vi "Read-Write Config File.vi"(0 "configuration file path":path=path "C:/ProgramData/PVI Systems/Vision Inspection System/Config.ini", 1 "Main Config in":T1 {"OPC Module Configs"."Data"."Variable Array"."status" items=["Good"=0, "Good_SubscriptionTransferred"=2949120, "Good_CompletesAsynchronously"=3014656, "Good_Overload"=3080192, "Good_Clamped"=3145728, "Good_LocalOverride"=9830400, "Good_EntryInserted"=10616832, "Good_EntryReplaced"=10682368, "Good_NoData"=10813440, "Good_MoreData"=10878976, "Good_CommunicationEvent"=10944512, "Good_ShutdownEvent"=11010048, "Good_CallAgain"=11075584, "Good_NonCriticalTimeout"=11141120, "Good_ResultsMayBeIncomplete"=12189696, "Good_DataIgnored"=14221312, "Uncertain"=1073741824, "Uncertain_ReferenceOutOfServer"=1080819712, "Uncertain_NoCommunicationLastUsableValue"=1083113472, "Uncertain_LastUsableValue"=1083179008, "Uncertain_SubstituteValue"=1083244544, "Uncertain_InitialValue"=1083310080, "Uncertain_SensorNotAccurate"=1083375616, "Uncertain_EngineeringUnitsExceeded"=1083441152, "Uncertain_SubNormal"=1083506688, "Uncertain_DataSubNormal"=1084489728, "Uncertain_ReferenceNotDeleted"=1086062592, "Uncertain_NotAllNodesAvailable"=1086324736, "Bad"=2147483648, "Bad_UnexpectedError"=2147549184, "Bad_InternalError"=2147614720, "Bad_OutOfMemory"=2147680256, "Bad_ResourceUnavailable"=2147745792, "Bad_CommunicationError"=2147811328, "Bad_EncodingError"=2147876864, "Bad_DecodingError"=2147942400, "Bad_EncodingLimitsExceeded"=2148007936, "Bad_UnknownResponse"=2148073472, "Bad_Timeout"=2148139008, "Bad_ServiceUnsupported"=2148204544, "Bad_Shutdown"=2148270080, "Bad_ServerNotConnected"=2148335616, "Bad_ServerHalted"=2148401152, "Bad_NothingToDo"=2148466688, "Bad_TooManyOperations"=2148532224, "Bad_DataTypeIdUnknown"=2148597760, "Bad_CertificateInvalid"=2148663296, "Bad_SecurityChecksFailed"=2148728832, "Bad_CertificateTimeInvalid"=2148794368, "Bad_CertificateIssuerTimeInvalid"=2148859904, "Bad_CertificateHostNameInvalid"=2148925440, "Bad_CertificateUriInvalid"=2148990976, "Bad_CertificateUseNotAllowed"=2149056512, "Bad_CertificateIssuerUseNotAllowed"=2149122048, "Bad_CertificateUntrusted"=2149187584, "Bad_CertificateRevocationUnknown"=2149253120, "Bad_CertificateIssuerRevocationUnknown"=2149318656, "Bad_CertificateRevoked"=2149384192, "Bad_CertificateIssuerRevoked"=2149449728, "Bad_UserAccessDenied"=2149515264, "Bad_IdentityTokenInvalid"=2149580800, "Bad_IdentityTokenRejected"=2149646336, "Bad_SecureChannelIdInvalid"=2149711872, "Bad_InvalidTimestamp"=2149777408, "Bad_NonceInvalid"=2149842944, "Bad_SessionIdInvalid"=2149908480, "Bad_SessionClosed"=2149974016, "Bad_SessionNotActivated"=2150039552, "Bad_SubscriptionIdInvalid"=2150105088, "Bad_RequestHeaderInvalid"=2150236160, "Bad_TimestampsToReturnInvalid"=2150301696, "Bad_RequestCancelledByClient"=2150367232, "Bad_NoCommunication"=2150694912, "Bad_WaitingForInitialData"=2150760448, "Bad_NodeIdInvalid"=2150825984, "Bad_NodeIdUnknown"=2150891520, "Bad_AttributeIdInvalid"=2150957056, "Bad_IndexRangeInvalid"=2151022592, "Bad_IndexRangeNoData"=2151088128, "Bad_DataEncodingInvalid"=2151153664, "Bad_DataEncodingUnsupported"=2151219200, "Bad_NotReadable"=2151284736, "Bad_NotWritable"=2151350272, "Bad_OutOfRange"=2151415808, "Bad_NotSupported"=2151481344, "Bad_NotFound"=2151546880, "Bad_ObjectDeleted"=2151612416, "Bad_NotImplemented"=2151677952, "Bad_MonitoringModeInvalid"=2151743488, "Bad_MonitoredItemIdInvalid"=2151809024, "Bad_MonitoredItemFilterInvalid"=2151874560, "Bad_MonitoredItemFilterUnsupported"=2151940096, "Bad_FilterNotAllowed"=2152005632, "Bad_StructureMissing"=2152071168, "Bad_EventFilterInvalid"=2152136704, "Bad_ContentFilterInvalid"=2152202240, "Bad_FilterOperandInvalid"=2152267776, "Bad_ContinuationPointInvalid"=2152333312, "Bad_NoContinuationPoints"=2152398848, "Bad_ReferenceTypeIdInvalid"=2152464384, "Bad_BrowseDirectionInvalid"=2152529920, "Bad_NodeNotInView"=2152595456, "Bad_ServerUriInvalid"=2152660992, "Bad_ServerNameMissing"=2152726528, "Bad_DiscoveryUrlMissing"=2152792064, "Bad_SempahoreFileMissing"=2152857600, "Bad_RequestTypeInvalid"=2152923136, "Bad_SecurityModeRejected"=2152988672, "Bad_SecurityPolicyRejected"=2153054208, "Bad_TooManySessions"=2153119744, "Bad_UserSignatureInvalid"=2153185280, "Bad_ApplicationSignatureInvalid"=2153250816, "Bad_NoValidCertificates"=2153316352, "Bad_RequestCancelledByRequest"=2153381888, "Bad_ParentNodeIdInvalid"=2153447424, "Bad_ReferenceNotAllowed"=2153512960, "Bad_NodeIdRejected"=2153578496, "Bad_NodeIdExists"=2153644032, "Bad_NodeClassInvalid"=2153709568, "Bad_BrowseNameInvalid"=2153775104, "Bad_BrowseNameDuplicated"=2153840640, "Bad_NodeAttributesInvalid"=2153906176, "Bad_TypeDefinitionInvalid"=2153971712, "Bad_SourceNodeIdInvalid"=2154037248, "Bad_TargetNodeIdInvalid"=2154102784, "Bad_DuplicateReferenceNotAllowed"=2154168320, "Bad_InvalidSelfReference"=2154233856, "Bad_ReferenceLocalOnly"=2154299392, "Bad_NoDeleteRights"=2154364928, "Bad_ServerIndexInvalid"=2154430464, "Bad_ViewIdUnknown"=2154496000, "Bad_TooManyMatches"=2154627072, "Bad_QueryTooComplex"=2154692608, "Bad_NoMatch"=2154758144, "Bad_MaxAgeInvalid"=2154823680, "Bad_HistoryOperationInvalid"=2154889216, "Bad_HistoryOperationUnsupported"=2154954752, "Bad_WriteNotSupported"=2155020288, "Bad_TypeMismatch"=2155085824, "Bad_MethodInvalid"=2155151360, "Bad_ArgumentsMissing"=2155216896, "Bad_TooManySubscriptions"=2155282432, "Bad_TooManyPublishRequests"=2155347968, "Bad_NoSubscription"=2155413504, "Bad_SequenceNumberUnknown"=2155479040, "Bad_MessageNotAvailable"=2155544576, "Bad_InsufficientClientProfile"=2155610112, "Bad_TcpServerTooBusy"=2155675648, "Bad_TcpMessageTypeInvalid"=2155741184, "Bad_TcpSecureChannelUnknown"=2155806720, "Bad_TcpMessageTooLarge"=2155872256, "Bad_TcpNotEnoughResources"=2155937792, "Bad_TcpInternalError"=2156003328, "Bad_TcpEndpointUrlInvalid"=2156068864, "Bad_RequestInterrupted"=2156134400, "Bad_RequestTimeout"=2156199936, "Bad_SecureChannelClosed"=2156265472, "Bad_SecureChannelTokenUnknown"=2156331008, "Bad_SequenceNumberInvalid"=2156396544, "Bad_ConfigurationError"=2156462080, "Bad_NotConnected"=2156527616, "Bad_DeviceFailure"=2156593152, "Bad_SensorFailure"=2156658688, "Bad_OutOfService"=2156724224, "Bad_DeadbandFilterInvalid"=2156789760, "Bad_RefreshInProgress"=2157379584, "Bad_ConditionAlreadyDisabled"=2157445120, "Bad_ConditionDisabled"=2157510656, "Bad_EventIdUnknown"=2157576192, "Bad_NoData"=2157641728, "Bad_DataLost"=2157772800, "Bad_DataUnavailable"=2157838336, "Bad_EntryExists"=2157903872, "Bad_NoEntryExists"=2157969408, "Bad_TimestampNotSupported"=2158034944, "Bad_InvalidArgument"=2158690304, "Bad_ConnectionRejected"=2158755840, "Bad_Disconnect"=2158821376, "Bad_ConnectionClosed"=2158886912, "Bad_InvalidState"=2158952448, "Bad_EndOfStream"=2159017984, "Bad_NoDataAvailable"=2159083520, "Bad_WaitingForResponse"=2159149056, "Bad_OperationAbandoned"=2159214592, "Bad_ExpectedStreamToBlock"=2159280128, "Bad_WouldBlock"=2159345664, "Bad_SyntaxError"=2159411200, "Bad_MaxConnectionsReached"=2159476736, "Bad_RequestTooLarge"=2159542272, "Bad_ResponseTooLarge"=2159607808, "Bad_EventNotAcknowledgeable"=2159738880, "Bad_InvalidTimestampArgument"=2159869952, "Bad_ProtocolVersionUnsupported"=2159935488, "Bad_StateNotActive"=2160001024, "Bad_FilterOperatorInvalid"=2160132096, "Bad_FilterOperatorUnsupported"=2160197632, "Bad_FilterOperandCountMismatch"=2160263168, "Bad_FilterElementInvalid"=2160328704, "Bad_FilterLiteralInvalid"=2160394240, "Bad_IdentityChangeNotSupported"=2160459776, "Bad_NotTypeDefinition"=2160590848, "Bad_ViewTimestampInvalid"=2160656384, "Bad_ViewParameterMismatch"=2160721920, "Bad_ViewVersionInvalid"=2160787456, "Bad_ConditionAlreadyEnabled"=2160852992, "Bad_DialogNotActive"=2160918528, "Bad_DialogResponseInvalid"=2160984064, "Bad_ConditionBranchAlreadyAcked"=2161049600, "Bad_ConditionBranchAlreadyConfirmed"=2161115136, "Bad_ConditionAlreadyShelved"=2161180672, "Bad_ConditionNotShelved"=2161246208, "Bad_ShelvingTimeOutOfRange"=2161311744, "Bad_AggregateListMismatch"=2161377280, "Bad_AggregateNotSupported"=2161442816, "Bad_AggregateInvalidInputs"=2161508352, "Bad_BoundNotFound"=2161573888, "Bad_BoundNotSupported"=2161639424, "Bad_AggregateConfigurationRejected"=2161770496, "Bad_TooManyMonitoredItems"=2161836032]; "PR Module Configs"."Settings"."PID 2 Parameters"."output range"."output low" format="%.2f"; "PR Module Configs"."Settings"."PID 2 Parameters"."output range"."output high" min=0.0 max=100.0 format="%.2f"; "PR Module Configs"."Settings"."PID 2 Parameters"."PID gains"."derivative time (Td, min)" format="%.3f"; "PR Module Configs"."Settings"."PID 2 Parameters"."PID gains"."integral time (Ti, min)" format="%.3f"; "PR Module Configs"."Settings"."PID 2 Parameters"."PID gains"."proportional gain (Kc)" format="%.3f"; "DO Module Configs"."Settings"."Valve Settings"."D-O Settings"."Output Channel" items=["Choose a Channel"]; "Steps"."Control" items=["Pump %", "Setpoint"]; "TCU Module Configs"."Settings"."Huber Unistat 410 Settings"."Address" min=0 max=99 format="%02.0f"; "TCU Module Configs"."Settings"."Julabo FP-50 Settings"."Pump Power" min=0 max=8 step=1; "TCU Module Configs"."Settings"."Lauda Settings"."Pump Power" min=0 max=8 step=1; "Flow Module Configs"."Settings"."Bronkhorst M14 Settings"."Smoothing Steps" min=1 step=1; "Flow Module Configs"."Settings"."Bronkhorst M13 Settings"."Smoothing Steps" min=1 step=1; "Pump Module Configs"."Settings"."Ismatech 3 Channel Settings"."Channel Number" min=0 max=3; "Pump Module Configs"."Settings"."Ismatech 3 Channel Settings"."Pump Number" min=1; "Pump Module Configs"."Settings"."ASIA Pump C"."channel" min=0 max=1 step=1; "Pump Module Configs"."Settings"."Masterflex"."Pump Number" min=1.0 max=20.0 step=1.0; "Pump Module Configs"."Settings"."Ismatech"."Pump Number" min=1.0 max=20.0 step=1.0; "Feed Module Configs"."Settings"."Bronkhorst M14 Settings"."Smoothing Steps" min=1 step=1; "Feed Module Configs"."Settings"."Ismatech 3 Channel Settings"."Channel Number" min=0 max=3; "Feed Module Configs"."Settings"."Ismatech 3 Channel Settings"."Pump Number" min=1; "Feed Module Configs"."Settings"."output range"."output low" min=0.0 max=100.0 format="%.2f"; "Feed Module Configs"."Settings"."output range"."output high" format="%.2f"; "Feed Module Configs"."Settings"."PID 2 Parameters"."PID gains"."derivative time (Td, min)" format="%.3f"; "Feed Module Configs"."Settings"."PID 2 Parameters"."PID gains"."integral time (Ti, min)" format="%.3f"; "Feed Module Configs"."Settings"."PID 2 Parameters"."PID gains"."proportional gain (Kc)" format="%.3f"; "Feed Module Configs"."Settings"."Bronkhorst M13 Flow Meter"."Smoothing Steps" min=1 step=1; "Feed Module Configs"."Settings"."ASIA Pump C"."channel" min=0 max=1 step=1; "Feed Module Configs"."Settings"."Ismatech"."Pump Number" min=1.0 max=20.0 step=1.0; "Feed Module Configs"."Settings"."Masterflex"."Pump Number" min=1.0 max=20.0 step=1.0}, 2 "Mode":T67=enum."Write", 3 "error in":errorcluster) -> (7 "Config File Path":path=path "C:/ProgramData/PVI Systems/Vision Inspection System/Config.ini", 8 "Main Config out":T1 {"OPC Module Configs"."Data"."Variable Array"."status" items=["Good"=0, "Good_SubscriptionTransferred"=2949120, "Good_CompletesAsynchronously"=3014656, "Good_Overload"=3080192, "Good_Clamped"=3145728, "Good_LocalOverride"=9830400, "Good_EntryInserted"=10616832, "Good_EntryReplaced"=10682368, "Good_NoData"=10813440, "Good_MoreData"=10878976, "Good_CommunicationEvent"=10944512, "Good_ShutdownEvent"=11010048, "Good_CallAgain"=11075584, "Good_NonCriticalTimeout"=11141120, "Good_ResultsMayBeIncomplete"=12189696, "Good_DataIgnored"=14221312, "Uncertain"=1073741824, "Uncertain_ReferenceOutOfServer"=1080819712, "Uncertain_NoCommunicationLastUsableValue"=1083113472, "Uncertain_LastUsableValue"=1083179008, "Uncertain_SubstituteValue"=1083244544, "Uncertain_InitialValue"=1083310080, "Uncertain_SensorNotAccurate"=1083375616, "Uncertain_EngineeringUnitsExceeded"=1083441152, "Uncertain_SubNormal"=1083506688, "Uncertain_DataSubNormal"=1084489728, "Uncertain_ReferenceNotDeleted"=1086062592, "Uncertain_NotAllNodesAvailable"=1086324736, "Bad"=2147483648, "Bad_UnexpectedError"=2147549184, "Bad_InternalError"=2147614720, "Bad_OutOfMemory"=2147680256, "Bad_ResourceUnavailable"=2147745792, "Bad_CommunicationError"=2147811328, "Bad_EncodingError"=2147876864, "Bad_DecodingError"=2147942400, "Bad_EncodingLimitsExceeded"=2148007936, "Bad_UnknownResponse"=2148073472, "Bad_Timeout"=2148139008, "Bad_ServiceUnsupported"=2148204544, "Bad_Shutdown"=2148270080, "Bad_ServerNotConnected"=2148335616, "Bad_ServerHalted"=2148401152, "Bad_NothingToDo"=2148466688, "Bad_TooManyOperations"=2148532224, "Bad_DataTypeIdUnknown"=2148597760, "Bad_CertificateInvalid"=2148663296, "Bad_SecurityChecksFailed"=2148728832, "Bad_CertificateTimeInvalid"=2148794368, "Bad_CertificateIssuerTimeInvalid"=2148859904, "Bad_CertificateHostNameInvalid"=2148925440, "Bad_CertificateUriInvalid"=2148990976, "Bad_CertificateUseNotAllowed"=2149056512, "Bad_CertificateIssuerUseNotAllowed"=2149122048, "Bad_CertificateUntrusted"=2149187584, "Bad_CertificateRevocationUnknown"=2149253120, "Bad_CertificateIssuerRevocationUnknown"=2149318656, "Bad_CertificateRevoked"=2149384192, "Bad_CertificateIssuerRevoked"=2149449728, "Bad_UserAccessDenied"=2149515264, "Bad_IdentityTokenInvalid"=2149580800, "Bad_IdentityTokenRejected"=2149646336, "Bad_SecureChannelIdInvalid"=2149711872, "Bad_InvalidTimestamp"=2149777408, "Bad_NonceInvalid"=2149842944, "Bad_SessionIdInvalid"=2149908480, "Bad_SessionClosed"=2149974016, "Bad_SessionNotActivated"=2150039552, "Bad_SubscriptionIdInvalid"=2150105088, "Bad_RequestHeaderInvalid"=2150236160, "Bad_TimestampsToReturnInvalid"=2150301696, "Bad_RequestCancelledByClient"=2150367232, "Bad_NoCommunication"=2150694912, "Bad_WaitingForInitialData"=2150760448, "Bad_NodeIdInvalid"=2150825984, "Bad_NodeIdUnknown"=2150891520, "Bad_AttributeIdInvalid"=2150957056, "Bad_IndexRangeInvalid"=2151022592, "Bad_IndexRangeNoData"=2151088128, "Bad_DataEncodingInvalid"=2151153664, "Bad_DataEncodingUnsupported"=2151219200, "Bad_NotReadable"=2151284736, "Bad_NotWritable"=2151350272, "Bad_OutOfRange"=2151415808, "Bad_NotSupported"=2151481344, "Bad_NotFound"=2151546880, "Bad_ObjectDeleted"=2151612416, "Bad_NotImplemented"=2151677952, "Bad_MonitoringModeInvalid"=2151743488, "Bad_MonitoredItemIdInvalid"=2151809024, "Bad_MonitoredItemFilterInvalid"=2151874560, "Bad_MonitoredItemFilterUnsupported"=2151940096, "Bad_FilterNotAllowed"=2152005632, "Bad_StructureMissing"=2152071168, "Bad_EventFilterInvalid"=2152136704, "Bad_ContentFilterInvalid"=2152202240, "Bad_FilterOperandInvalid"=2152267776, "Bad_ContinuationPointInvalid"=2152333312, "Bad_NoContinuationPoints"=2152398848, "Bad_ReferenceTypeIdInvalid"=2152464384, "Bad_BrowseDirectionInvalid"=2152529920, "Bad_NodeNotInView"=2152595456, "Bad_ServerUriInvalid"=2152660992, "Bad_ServerNameMissing"=2152726528, "Bad_DiscoveryUrlMissing"=2152792064, "Bad_SempahoreFileMissing"=2152857600, "Bad_RequestTypeInvalid"=2152923136, "Bad_SecurityModeRejected"=2152988672, "Bad_SecurityPolicyRejected"=2153054208, "Bad_TooManySessions"=2153119744, "Bad_UserSignatureInvalid"=2153185280, "Bad_ApplicationSignatureInvalid"=2153250816, "Bad_NoValidCertificates"=2153316352, "Bad_RequestCancelledByRequest"=2153381888, "Bad_ParentNodeIdInvalid"=2153447424, "Bad_ReferenceNotAllowed"=2153512960, "Bad_NodeIdRejected"=2153578496, "Bad_NodeIdExists"=2153644032, "Bad_NodeClassInvalid"=2153709568, "Bad_BrowseNameInvalid"=2153775104, "Bad_BrowseNameDuplicated"=2153840640, "Bad_NodeAttributesInvalid"=2153906176, "Bad_TypeDefinitionInvalid"=2153971712, "Bad_SourceNodeIdInvalid"=2154037248, "Bad_TargetNodeIdInvalid"=2154102784, "Bad_DuplicateReferenceNotAllowed"=2154168320, "Bad_InvalidSelfReference"=2154233856, "Bad_ReferenceLocalOnly"=2154299392, "Bad_NoDeleteRights"=2154364928, "Bad_ServerIndexInvalid"=2154430464, "Bad_ViewIdUnknown"=2154496000, "Bad_TooManyMatches"=2154627072, "Bad_QueryTooComplex"=2154692608, "Bad_NoMatch"=2154758144, "Bad_MaxAgeInvalid"=2154823680, "Bad_HistoryOperationInvalid"=2154889216, "Bad_HistoryOperationUnsupported"=2154954752, "Bad_WriteNotSupported"=2155020288, "Bad_TypeMismatch"=2155085824, "Bad_MethodInvalid"=2155151360, "Bad_ArgumentsMissing"=2155216896, "Bad_TooManySubscriptions"=2155282432, "Bad_TooManyPublishRequests"=2155347968, "Bad_NoSubscription"=2155413504, "Bad_SequenceNumberUnknown"=2155479040, "Bad_MessageNotAvailable"=2155544576, "Bad_InsufficientClientProfile"=2155610112, "Bad_TcpServerTooBusy"=2155675648, "Bad_TcpMessageTypeInvalid"=2155741184, "Bad_TcpSecureChannelUnknown"=2155806720, "Bad_TcpMessageTooLarge"=2155872256, "Bad_TcpNotEnoughResources"=2155937792, "Bad_TcpInternalError"=2156003328, "Bad_TcpEndpointUrlInvalid"=2156068864, "Bad_RequestInterrupted"=2156134400, "Bad_RequestTimeout"=2156199936, "Bad_SecureChannelClosed"=2156265472, "Bad_SecureChannelTokenUnknown"=2156331008, "Bad_SequenceNumberInvalid"=2156396544, "Bad_ConfigurationError"=2156462080, "Bad_NotConnected"=2156527616, "Bad_DeviceFailure"=2156593152, "Bad_SensorFailure"=2156658688, "Bad_OutOfService"=2156724224, "Bad_DeadbandFilterInvalid"=2156789760, "Bad_RefreshInProgress"=2157379584, "Bad_ConditionAlreadyDisabled"=2157445120, "Bad_ConditionDisabled"=2157510656, "Bad_EventIdUnknown"=2157576192, "Bad_NoData"=2157641728, "Bad_DataLost"=2157772800, "Bad_DataUnavailable"=2157838336, "Bad_EntryExists"=2157903872, "Bad_NoEntryExists"=2157969408, "Bad_TimestampNotSupported"=2158034944, "Bad_InvalidArgument"=2158690304, "Bad_ConnectionRejected"=2158755840, "Bad_Disconnect"=2158821376, "Bad_ConnectionClosed"=2158886912, "Bad_InvalidState"=2158952448, "Bad_EndOfStream"=2159017984, "Bad_NoDataAvailable"=2159083520, "Bad_WaitingForResponse"=2159149056, "Bad_OperationAbandoned"=2159214592, "Bad_ExpectedStreamToBlock"=2159280128, "Bad_WouldBlock"=2159345664, "Bad_SyntaxError"=2159411200, "Bad_MaxConnectionsReached"=2159476736, "Bad_RequestTooLarge"=2159542272, "Bad_ResponseTooLarge"=2159607808, "Bad_EventNotAcknowledgeable"=2159738880, "Bad_InvalidTimestampArgument"=2159869952, "Bad_ProtocolVersionUnsupported"=2159935488, "Bad_StateNotActive"=2160001024, "Bad_FilterOperatorInvalid"=2160132096, "Bad_FilterOperatorUnsupported"=2160197632, "Bad_FilterOperandCountMismatch"=2160263168, "Bad_FilterElementInvalid"=2160328704, "Bad_FilterLiteralInvalid"=2160394240, "Bad_IdentityChangeNotSupported"=2160459776, "Bad_NotTypeDefinition"=2160590848, "Bad_ViewTimestampInvalid"=2160656384, "Bad_ViewParameterMismatch"=2160721920, "Bad_ViewVersionInvalid"=2160787456, "Bad_ConditionAlreadyEnabled"=2160852992, "Bad_DialogNotActive"=2160918528, "Bad_DialogResponseInvalid"=2160984064, "Bad_ConditionBranchAlreadyAcked"=2161049600, "Bad_ConditionBranchAlreadyConfirmed"=2161115136, "Bad_ConditionAlreadyShelved"=2161180672, "Bad_ConditionNotShelved"=2161246208, "Bad_ShelvingTimeOutOfRange"=2161311744, "Bad_AggregateListMismatch"=2161377280, "Bad_AggregateNotSupported"=2161442816, "Bad_AggregateInvalidInputs"=2161508352, "Bad_BoundNotFound"=2161573888, "Bad_BoundNotSupported"=2161639424, "Bad_AggregateConfigurationRejected"=2161770496, "Bad_TooManyMonitoredItems"=2161836032]; "PR Module Configs"."Settings"."PID 2 Parameters"."output range"."output low" format="%.2f"; "PR Module Configs"."Settings"."PID 2 Parameters"."output range"."output high" min=0.0 max=100.0 format="%.2f"; "PR Module Configs"."Settings"."PID 2 Parameters"."PID gains"."derivative time (Td, min)" format="%.3f"; "PR Module Configs"."Settings"."PID 2 Parameters"."PID gains"."integral time (Ti, min)" format="%.3f"; "PR Module Configs"."Settings"."PID 2 Parameters"."PID gains"."proportional gain (Kc)" format="%.3f"; "DO Module Configs"."Settings"."Valve Settings"."D-O Settings"."Output Channel" items=["Choose a Channel"]; "Steps"."Control" items=["Pump %", "Setpoint"]; "TCU Module Configs"."Settings"."Huber Unistat 410 Settings"."Address" min=0 max=99 format="%02.0f"; "TCU Module Configs"."Settings"."Julabo FP-50 Settings"."Pump Power" min=0 max=8 step=1; "TCU Module Configs"."Settings"."Lauda Settings"."Pump Power" min=0 max=8 step=1; "Flow Module Configs"."Settings"."Bronkhorst M14 Settings"."Smoothing Steps" min=1 step=1; "Flow Module Configs"."Settings"."Bronkhorst M13 Settings"."Smoothing Steps" min=1 step=1; "Pump Module Configs"."Settings"."Ismatech 3 Channel Settings"."Channel Number" min=0 max=3; "Pump Module Configs"."Settings"."Ismatech 3 Channel Settings"."Pump Number" min=1; "Pump Module Configs"."Settings"."ASIA Pump C"."channel" min=0 max=1 step=1; "Pump Module Configs"."Settings"."Masterflex"."Pump Number" min=1.0 max=20.0 step=1.0; "Pump Module Configs"."Settings"."Ismatech"."Pump Number" min=1.0 max=20.0 step=1.0; "Feed Module Configs"."Settings"."Bronkhorst M14 Settings"."Smoothing Steps" min=1 step=1; "Feed Module Configs"."Settings"."Ismatech 3 Channel Settings"."Channel Number" min=0 max=3; "Feed Module Configs"."Settings"."Ismatech 3 Channel Settings"."Pump Number" min=1; "Feed Module Configs"."Settings"."output range"."output low" min=0.0 max=100.0 format="%.2f"; "Feed Module Configs"."Settings"."output range"."output high" format="%.2f"; "Feed Module Configs"."Settings"."PID 2 Parameters"."PID gains"."derivative time (Td, min)" format="%.3f"; "Feed Module Configs"."Settings"."PID 2 Parameters"."PID gains"."integral time (Ti, min)" format="%.3f"; "Feed Module Configs"."Settings"."PID 2 Parameters"."PID gains"."proportional gain (Kc)" format="%.3f"; "Feed Module Configs"."Settings"."Bronkhorst M13 Flow Meter"."Smoothing Steps" min=1 step=1; "Feed Module Configs"."Settings"."ASIA Pump C"."channel" min=0 max=1 step=1; "Feed Module Configs"."Settings"."Ismatech"."Pump Number" min=1.0 max=20.0 step=1.0; "Feed Module Configs"."Settings"."Masterflex"."Pump Number" min=1.0 max=20.0 step=1.0}, 10 "error out":errorcluster)   [LabVIEW 2018, in "Config Module.lvlib"]
uses:
  Config Module.lvlib
  Controls/Config File Operation Enum.ctl
  Controls/Main Config Cluster.ctl
  OPC/OPC Module Config.ctl
  Scale Module Folder/Measure Instrument/State Enum.ctl
  <vilib>/Utility/miscctls.llb/LVPoint32TypeDef.ctl
  OPC/OPC Settings.ctl
  OPC/Variable Data Cluster.ctl
  <vilib>/OPCUA/controls/NodeId.ctl
  <vilib>/OPCUA/controls/OPC UA StatusCode.ctl
  <vilib>/OPCUA/controls/Subscription ID.ctl
  <vilib>/OPCUA/controls/OPC UA Client Refnum.ctl
  <vilib>/OPCUA/controls/Subscription Data Change.ctl
  <vilib>/OPCUA/controls/Data Type.ctl
  OPC/OPC Tag Data.ctl
  Feed Module/Controls/Feed Module Config Cluster.ctl
  Feed Module/Controls/Feed Module Settings Cluster.ctl
  Ismatec ISM 831C/Controls/Ismatech ISM831C Settings Cluster.ctl
  Masterflex 7550-30/Controls/Settings Cluster.ctl
  Mettler Toledo/Controls/Settings Cluster.ctl
  Bronkhorst M13 Flow Meter/Settings Cluster.ctl
  Measure Instrument/PID 2 Parameters Cluster.ctl
  Measure Instrument/PID Input Enum.ctl
  Measure Instrument/PID 2 Output Enum.ctl
  Tacmina QI/Tacmina QI DAQ Setting.ctl
  KNF Pump/Settings Cluster plus SIMDOS.ctl
  ASIA Pump/Pump Settings.ctl
  VICI M50 Party Mode/Settings Cluster.ctl
  FLOM Pump/Settings Cluster.ctl
  SSI PR Class/SSI PR or LD Settings Cluster.ctl
  Masterflex 75211/Masterflex 75211 DAQ Setting.ctl
  SSI PR Class/SSI P40 Settings Cluster.ctl
  Ismatec 78001/Ismatec 4083.ctl
  Bronkhorst M14 Flow Meter/Settings Cluster.ctl
  TT Module/Controls/TT Module Config Cluster.ctl
  Tag VIs/Numeric Alarm Settings Cluster.ctl
  Acquisition/Hardware Configuration.ctl
  Acquisition/Task Cluster.ctl
  PT Module/Controls/PT Module Config Cluster.ctl
  Scale Module Folder/Feed Module/Controls/Scale Module Config Cluster.ctl
  Scale Module Folder/Feed Module/Controls/Scale Module Settings Cluster.ctl
  Pump Module Folder/Pump Module Config Cluster.ctl
  Pump Module Folder/Pump Module Settings Cluster.ctl
  LabJack Module/Controls/U3 Module Config Cluster.ctl
  Decoration Module/Decoration Module Config Cluster.ctl
  Flow Module Folder/Feed Module/Controls/Flow Module Config Cluster.ctl
  Flow Module Folder/Feed Module/Controls/Flow Module Settings Cluster.ctl
  TCU Module/TCU Module Folder/TCU Module Config Cluster.ctl
  TCU Module/TCU Module Folder/TCU Module Settings Cluster.ctl
  TCU Module/TCU Module Folder/Measure Instrument/Output Devices.ctl
  Huber TCU/Huber Settings.ctl
  Lauda Integral XT-150 TCU/Lauda Settings.ctl
  Julabo Type 1 TCU/Julabo Type 1 TCU Folder/Julabo FP-50 Settings.ctl
  Huber Unistat 410 TCU/Huber Unistat 410 RS485 Settings.ctl
  D-O Module Folder/Not Sure Where this is Used.ctl
  Sequencing/Squence Control.ctl
  D-O Module Folder/D-O Module Config Cluster.ctl
  D-O Module Folder/Valve Clusters.ctl
  D-O Module Folder/D-O Module Settings Cluster.ctl
  D-O Module Folder/D-O Device Settings Cluster.ctl
  VICI Electronic Actuator/VICI Electronic Actuator Settings.ctl
  Pressure Regulator Control Module/Pressure Regulator/Controls/4-20mA Module Config Cluster.ctl
  Pressure Regulator Control Module/Pressure Regulator/Controls/4-20mA Module Settings Cluster.ctl
  Pressure Transmitter/Pressure Transmitter Device Settings.ctl
  Pressure Reg Module/Pressure Regulator Device Settings.ctl
  Sonicator Module Folder/Feed Module/Controls/Sonicator Module Config Cluster.ctl
  Sonicator Module Folder/Feed Module/Controls/Sonicator Module Settings Cluster.ctl
  Sonic Systems P100/Sonic Systems P100 Settings.ctl
  Agitator Module Folder - Copy/Feed Module/Controls/Agitator Module Config Cluster.ctl
  Agitator Module Folder - Copy/Feed Module/Controls/Agitator Module Settings Cluster.ctl
  XML Config/XML Config.lvlib
  TT Module/TT Module.lvlib
  Feed Module/Feed Module.lvlib
  Ismatec ISM 831C/Ismatec ISM 831C.lvlib
  Masterflex 7550-30/Masterflex 7550-30.lvlib
  Mettler Toledo/Mettler Toledo.lvlib
  Bronkhorst M13 Flow Meter/Bronkhorst M13 Flow Meter.lvlib
  DAQ/DAQ.lvlib
  PT Module/PT Module.lvlib
  Scale Module Folder/Scale Module.lvlib
  Pump Module Folder/Pump Module.lvlib
  LabJack Module/U3 Module.lvlib
  Flow Module Folder/Flow Module.lvlib
  Tacmina QI/Tacmina QI.lvlib
  KNF Pump/KNF SIMDOS.lvlib
  Huber TCU/Huber Ministat 230 TCU.lvlib
  TCU Module/TCU Module Folder/TCU Module.lvlib
  Lauda Integral XT-150 TCU/Lauda TCU.lvlib
  Julabo Type 1 TCU/Julabo Type 1 TCU Folder/Julabo Type FP-50 TCU.lvlib
  ASIA Pump.lvlib
  Sequencing/Sequencing Library.lvlib
  VICI M50 Party Mode/VICI M6 M50 Party Mode.lvlib
  D-O Module Folder/D-O Module.lvlib
  Pressure Transmitter/Pressure Transmitter Library.lvlib
  Pressure Regulator Control Module/Pressure Regulator/4-20mA Module.lvlib
  Pressure Reg Module/Pressure Regulator Library.lvlib
  FLOM Pump/FLOM Pump.lvlib
  SSI PR Class/SSI PR or LD Pump.lvlib
  OPC/OPC UA.lvlib
  Scale Module Folder/Measure Instrument/Scale Module Engine.lvlib
  D-O Module Folder/DIO Valve/VICI Electronic Actuator.lvlib
  Masterflex 75211/Masterflex 75211.lvlib
  SSI PR Class/SSI P40 Pump.lvlib
  Huber Unistat 410 TCU/Huber Unistat 410 TCU.lvlib
  Ismatec 78001/Ismatec 4308.lvlib
  Bronkhorst M14 Flow Meter/Bronkhorst M14 Flow Meter.lvlib
  Sonicator Module Folder/Sonicator Module.lvlib
  Sonic Systems P100/Sonic Systems P100.lvlib
  Agitator Module Folder - Copy/Agitator Module.lvlib
panel:
  # "Agitator Settings"
  # "Sonicator Settings"
  # "Instrument Settings"
  # "Instrument Settings"
  # "Output Instruments"
  # "Flow Meter Settings"
  # "Output Instruments"
  # "Scale Settings"
  # "Output Instruments"
  # "Input Instruments"
  # "Agitator Settings"
  # "Sonicator Settings"
  # "Instrument Settings"
  # "Instrument Settings"
  # "Output Instruments"
  # "Flow Meter Settings"
  # "Output Instruments"
  # "Scale Settings"
  # "Output Instruments"
  # "Input Instruments"
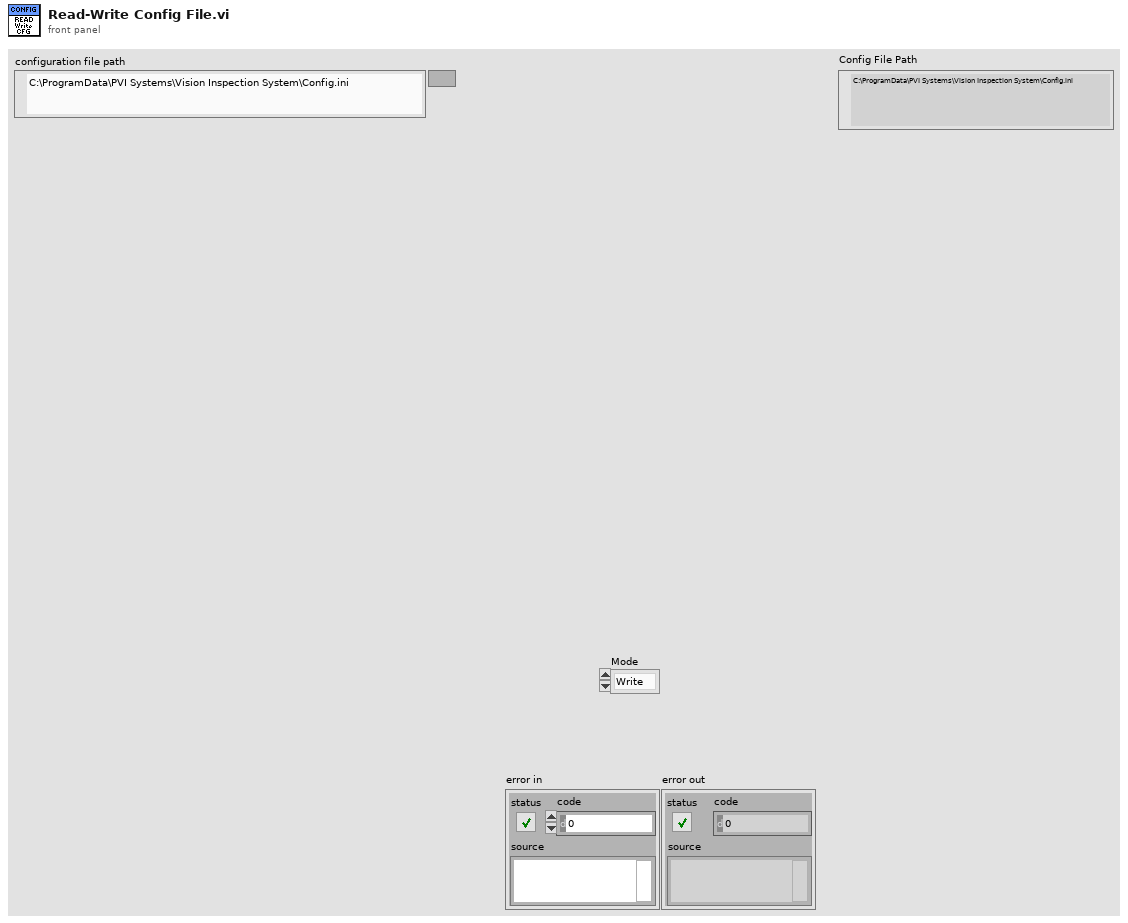
[diagram p1: front panel]
types:
  T1 = typedef "Config Module.lvlib/Main Config Cluster.ctl" = cluster{"Notebook":string, "OPC Module Configs":T2[], "Feed Module Configs":T12[], "Log File Path":path, "TT Module Configs":T31[], "DAQ Config":T33, "PT Module Configs":T35[], "Scale Module Configs":T36[], "Pump Module Configs":T38[], "U3 Module Configs":T40[], "Decoration Module Configs":T41[], "Flow Module Configs":T42[], "TCU Module Configs":T44[], "Steps":T51, "Abort":bool, "DO Module Configs":T53[], "PR Module Configs":T58[], "SC Module Configs":T62[], "AM Module Configs":T65[], "Cycle Period":dbl}
  T2 = typedef "OPC UA.lvlib/OPC Module Config.ctl" = cluster{"State":T3, "GUID":string, "Drop Coords":T4, "Configuration":T5, "First Iteration":bool, "Data":cluster{"Object Name":string, "Variable Array":T6[]}[], "Process Name":string, "Load Count":i32, "Log Started":bool, "subscription ID out":T9, "OPC UA client refnum out":T10, "Event Registration Refnum":refnum<event-registration>, "Start Time":timestamp, "Current Time":timestamp, "Tag Data":T11[]}
  T3 = typedef "Scale Module.lvlib/Scale Module Engine.lvlib/State Enum.ctl" = enum16{"Measuring", "Idle"}
  T4 = typedef "LVPoint32TypeDef.ctl" = cluster{"Horizontal":i32, "Vertical":i32}
  T5 = typedef "OPC UA.lvlib/OPC Settings.ctl" = cluster{"Cycle Period":dbl, "server endpoint URL":string, "security policy":cluster{"message mode":enum16{"None", "Sign", "Sign and Encrypt"}, "security":enum16{"Basic256", "Basic128Rsa15"}}, "Trust Any Server":bool}
  T6 = typedef "OPC UA.lvlib/Variable Data Cluster.ctl" = cluster{"node ID":T7, "browse name":string, "status":T8, "timestamp":timestamp, "value ":variant}
  T7 = typedef "NodeId.ctl" = string
  T8 = typedef "OPC UA StatusCode.ctl" = u32
  T9 = typedef "Subscription ID.ctl" = u32
  T10 = typedef "OPC UA Client Refnum.ctl" = refnum<k21>
  T11 = typedef "OPC UA.lvlib/OPC Tag Data.ctl" = cluster{"Include this Device":bool, "Device Name":string, "OPC Tag Data":cluster{"Tag":string, "Value":variant, "Time Stamp":timestamp}[]}
  T12 = typedef "Feed Module.lvlib/Feed Module Config Cluster.ctl" = cluster{"GUID":string, "Drop Coords":T4, "Process Name":string, "Queue Name":string, "Settings":T13, "Settings Load Count":i32, "OP Load Count":i32}
  T13 = typedef "Feed Module.lvlib/Feed Module Settings Cluster.ctl" = cluster{"Cycle Period":dbl, "Ismatech":T14, "Masterflex":T15, "Mettler":T16, "Bronkhorst M13 Flow Meter":T17, "PID 2 Parameters":T18, "Manual Entry":dbl, "Auto?":bool, "output range":cluster{"output high":dbl, "output low":dbl}, "Tacmina Settings":T21, "KNF SIMDOS Settings":T22, "ASIA Pump C":T23, "VICI Settings":T24, "FLOM Settings":T25, "SSI PR/LD Settings":T26, "Masterflex 75211 Settings":T27, "SSI P40 Settings":T28, "Ismatech 3 Channel Settings":T29, "Bronkhorst M14 Settings":T30}
  T14 = typedef "Ismatec ISM 831C.lvlib/Ismatech ISM831C Settings Cluster.ctl" = cluster{"VISA resource name":refnum<visa-resource-name>, "Simulated?":bool, "Pump Number":dbl, "Reverse?":bool}
  T15 = typedef "Masterflex 7550-30.lvlib/Settings Cluster.ctl" = cluster{"VISA resource name":refnum<visa-resource-name>, "Simulated?":bool, "Pump Number":dbl, "Reverse?":bool}
  T16 = typedef "Mettler Toledo.lvlib/Settings Cluster.ctl" = cluster{"VISA resource name":refnum<visa-resource-name>, "Simulated?":bool}
  T17 = typedef "Bronkhorst M13 Flow Meter.lvlib/Settings Cluster.ctl" = cluster{"VISA resource name":refnum<visa-resource-name>, "Simulated?":bool, "Smoothing Steps":i32}
  T18 = typedef "PID 2 Parameters Cluster.ctl" = cluster{"Input Device":T19, "Output Device":T20, "Setpoint":dbl, "PID gains":cluster{"proportional gain (Kc)":dbl, "integral time (Ti, min)":dbl, "derivative time (Td, min)":dbl}}
  T19 = typedef "PID Input Enum.ctl" = enum16{"Default", "Bronkhorst M13", "Bronkhorst M14", "Scale Rate of Change"}
  T20 = typedef "PID 2 Output Enum.ctl" = enum16{"Default", "Ismatec ISM 4308", "Ismatec ISM 831C", "Masterflex 7550-30", "VICI", "Tacmina QI", "KNF SIMDOS", "ASIA Type C", "FLOM UI-22-11", "SSI PR/LD", "SSI P40", "Masterflex 75211-70"}
  T21 = typedef "Tacmina QI.lvlib/Tacmina QI DAQ Setting.ctl" = cluster{"Analog DAQ Task":refnum<k21>, "Digital DAQ Task":refnum<k21>}
  T22 = typedef "KNF SIMDOS.lvlib/Settings Cluster plus SIMDOS.ctl" = cluster{"VISA resource name":refnum<visa-resource-name>, "Simulated?":bool}
  T23 = typedef "ASIA Pump.lvlib/Pump Settings.ctl" = cluster{"ASIA Pump #":i32, "channel":i32, "Simulated":bool}
  T24 = typedef "VICI M6 M50 Party Mode.lvlib/Settings Cluster.ctl" = cluster{"VISA resource name":refnum<visa-resource-name>, "Simulated?":bool, "Pump Letter":string, "Reverse?":bool}
  T25 = typedef "FLOM Pump.lvlib/Settings Cluster.ctl" = cluster{"VISA resource name":refnum<visa-resource-name>, "Simulated?":bool, "Pump Number":dbl}
  T26 = typedef "SSI PR or LD Pump.lvlib/SSI PR or LD Settings Cluster.ctl" = cluster{"VISA resource name":refnum<visa-resource-name>, "Simulated?":bool}
  T27 = typedef "Masterflex 75211.lvlib/Masterflex 75211 DAQ Setting.ctl" = cluster{"Analog DAQ Task":refnum<k21>, "Digital DAQ Task":refnum<k21>}
  T28 = typedef "SSI P40 Pump.lvlib/SSI P40 Settings Cluster.ctl" = cluster{"VISA resource name":refnum<visa-resource-name>, "Simulated?":bool}
  T29 = typedef "Ismatec 4308.lvlib/Ismatec 4083.ctl" = cluster{"VISA resource name":refnum<visa-resource-name>, "Pump Number":i16, "Channel Number":i16, "Simulated?":bool, "Reverse?":bool}
  T30 = typedef "Bronkhorst M14 Flow Meter.lvlib/Settings Cluster.ctl" = cluster{"VISA resource name":refnum<visa-resource-name>, "Simulated?":bool, "Smoothing Steps":i32}
  T31 = typedef "TT Module.lvlib/TT Module Config Cluster.ctl" = cluster{"GUID":string, "Drop Coords":T4, "Input Channel Tag Name ":string, "Process Name":string, "Queue Name":string, "Input Channel Numeric Alarm Settings":T32[]}
  T32 = typedef "Numeric Alarm Settings Cluster.ctl" = cluster{"enable? (F)":bool, "name":string, "alarm type":enum16{"HI_HI", "HI", "LO", "LO_LO"}, "level/change":dbl, "deadband/time":dbl, "alarm delay":dbl, "priority":u32, "ack type":enum16{"Auto", "User", "None", "Each Occurrence"}, "area":string, "description":string, "log? (T)":bool}
  T33 = typedef "DAQ.lvlib/Hardware Configuration.ctl" = cluster{"Tasks":T34[]}
  T34 = typedef "Task Cluster.ctl" = cluster{"DAQmx Task":refnum<k21>, "Read-Write Radio":enum32{"Read", "Write"}}
  T35 = typedef "PT Module.lvlib/PT Module Config Cluster.ctl" = cluster{"GUID":string, "Drop Coords":T4, "Input Channel Tag Name ":string, "Process Name":string, "Queue Name":string, "Input Channel Numeric Alarm Settings":T32[]}
  T36 = typedef "Scale Module.lvlib/Scale Module Config Cluster.ctl" = cluster{"GUID":string, "Drop Coords":T4, "Process Name":string, "Queue Name":string, "Settings":T37, "Load Count":i32}
  T37 = typedef "Scale Module.lvlib/Scale Module Settings Cluster.ctl" = cluster{"Cycle Period":dbl, "Mettler":T16, "Scale Type":string}
  T38 = typedef "Pump Module.lvlib/Pump Module Config Cluster.ctl" = cluster{"GUID":string, "Drop Coords":T4, "Process Name":string, "Queue Name":string, "Settings":T39, "Load Count":i32}
  T39 = typedef "Pump Module.lvlib/Pump Module Settings Cluster.ctl" = cluster{"Cycle Period":dbl, "Manual Entry":dbl, "Output Device":T20, "Ismatech":T14, "Ismatech 3 Channel Settings":T29, "Masterflex":T15, "VICI Settings":T24, "Tacmina Settings":T21, "KNF SIMDOS Settings":T22, "ASIA Pump C":T23, "FLOM Settings":T25, "SSI PR/LD Settings":T26, "SSI P40 Settings":T26, "Masterflex 75211 Settings":T27, "Pump Calibration File":path, "Calibration Slope":dbl, "Calibration Y Intercept":dbl, "Pump Cal Enum":u16}
  T40 = typedef "U3 Module.lvlib/U3 Module Config Cluster.ctl" = cluster{"GUID":string, "Drop Coords":T4, "AI Channel Number":enum16{"Default", "AI0", "AI1", "AI2", "AI3", "AI4", "AI5", "AI6", "AI7"}, "Process Name":string, "Queue Name":string, "Input Channel Numeric Alarm Settings":T32[]}
  T41 = typedef "Decoration Module Config Cluster.ctl" = cluster{"GUID":string, "Drop Coords":T4, "Decoration Filepath":path}
  T42 = typedef "Flow Module.lvlib/Flow Module Config Cluster.ctl" = cluster{"GUID":string, "Drop Coords":T4, "Process Name":string, "Queue Name":string, "Settings":T43, "Load Count":i32}
  T43 = typedef "Flow Module.lvlib/Flow Module Settings Cluster.ctl" = cluster{"Cycle Period":dbl, "Flow Meter Type":string, "Bronkhorst M13 Settings":T17, "Bronkhorst M14 Settings":T30}
  T44 = typedef "TCU Module.lvlib/TCU Module Config Cluster.ctl" = cluster{"GUID":string, "Drop Coords":T4, "Process Name":string, "Queue Name":string, "Settings":T45, "Load Count":i32, "Power Level Changed":bool}
  T45 = typedef "TCU Module.lvlib/TCU Module Settings Cluster.ctl" = cluster{"Cycle Period":dbl, "Setpoint Entry":dbl, "Output Device":T46, "Huber Ministat 230 Settings":T47, "Lauda Settings":T48, "Julabo FP-50 Settings":T49, "Internal Control?":bool, "Huber Unistat 410 Settings":T50}
  T46 = typedef "Output Devices.ctl" = enum16{"Default", "Huber Ministat 230", "Huber Unistat 410", "Lauda XT-150", "Julabo FP-50"}
  T47 = typedef "Huber Ministat 230 TCU.lvlib/Huber Settings.ctl" = cluster{"VISA resource name":refnum<visa-resource-name>, "Simulated?":bool}
  T48 = typedef "Lauda TCU.lvlib/Lauda Settings.ctl" = cluster{"VISA resource name":refnum<visa-resource-name>, "Simulated?":bool, "Pump Power":i32}
  T49 = typedef "Julabo Type FP-50 TCU.lvlib/Julabo FP-50 Settings.ctl" = cluster{"VISA resource name":refnum<visa-resource-name>, "Simulated?":bool, "Pump Power":i32}
  T50 = typedef "Huber Unistat 410 TCU.lvlib/Huber Unistat 410 RS485 Settings.ctl" = cluster{"VISA resource name":refnum<visa-resource-name>, "Address":i8, "Simulated?":bool}
  T51 = typedef "Not Sure Where this is Used.ctl" = T52[]
  T52 = typedef "Sequencing Library.lvlib/Squence Control.ctl" = cluster{"Module":string, "Control":u16, "Value":dbl, "Wait (sec)":dbl}
  T53 = typedef "D-O Module.lvlib/D-O Module Config Cluster.ctl" = cluster{"GUID":string, "Drop Coords":T4, "Process Name":string, "Queue Name":string, "Settings":T54, "Load Count":i32}
  T54 = typedef "D-O Module.lvlib/Valve Clusters.ctl" = cluster{"Valve Settings":T55, "Valve Type":enum16{"Default", "Digital Output Valve", "VICI Electronic Actuator"}, "Time On (Sec)":dbl, "Time Off (Sec)":dbl, "Run?":bool}
  T55 = typedef "D-O Module.lvlib/D-O Module Settings Cluster.ctl" = cluster{"D-O Settings":T56, "VICI Electronic Actuator":T57}
  T56 = typedef "D-O Module.lvlib/D-O Device Settings Cluster.ctl" = cluster{"DAQmx Task Name":refnum<k21>, "Output Channel":u16, "Output Channel Names":string[]}
  T57 = typedef "VICI Electronic Actuator.lvlib/VICI Electronic Actuator Settings.ctl" = cluster{"VISA resource name":refnum<visa-resource-name>, "Mode":enum16{"Two Positions With Stops", "Two Positions Without Stops", "Mutiposition"}, "Simulated":bool}
  T58 = typedef "4-20mA Module.lvlib/4-20mA Module Config Cluster.ctl" = cluster{"GUID":string, "Drop Coords":T4, "Process Name":string, "Queue Name":string, "Settings":T59, "Settings Load Count":i32}
  T59 = typedef "4-20mA Module.lvlib/4-20mA Module Settings Cluster.ctl" = cluster{"Cycle Period":dbl, "PID 2 Parameters":cluster{"Input Device":enum16{"Default", "4-20mA"}, "Output Device":enum16{"Default", "Equilibar Pressure Reg", "Flow Regulator"}, "Setpoint":dbl, "PID gains":cluster{"proportional gain (Kc)":dbl, "integral time (Ti, min)":dbl, "derivative time (Td, min)":dbl}, "output range":cluster{"output low":dbl, "output high":dbl}}, "Manual Entry":dbl, "Auto?":bool, "4-20mA Input Settings":T60, "4-20mA Out Settings":T61, "Input Channel Tag Name ":string}
  T60 = typedef "Pressure Transmitter Library.lvlib/Pressure Transmitter Device Settings.ctl" = cluster{"Input Channel ":u16}
  T61 = typedef "Pressure Regulator Library.lvlib/Pressure Regulator Device Settings.ctl" = cluster{"Output DAQ Task":refnum<k21>}
  T62 = typedef "Sonicator Module.lvlib/Sonicator Module Config Cluster.ctl" = cluster{"GUID":string, "Drop Coords":T4, "Process Name":string, "Queue Name":string, "Settings":T63, "Load Count":i32}
  T63 = typedef "Sonicator Module.lvlib/Sonicator Module Settings Cluster.ctl" = cluster{"Cycle Period":dbl, "Sonicator Type":string, "SS P100 Settings":T64, "Setpoint (µm)":dbl, "Cutoff (µm)":dbl}
  T64 = typedef "Sonic Systems P100.lvlib/Sonic Systems P100 Settings.ctl" = cluster{"VISA resource name":refnum<visa-resource-name>, "Simulated?":bool}
  T65 = typedef "Agitator Module.lvlib/Agitator Module Config Cluster.ctl" = cluster{"GUID":string, "Drop Coords":T4, "Process Name":string, "Queue Name":string, "Settings":T66, "Load Count":i32}
  T66 = typedef "Agitator Module.lvlib/Agitator Module Settings Cluster.ctl" = cluster{"Cycle Period":dbl, "Agitator Type":string, "Setpoint (µm)":dbl}
  T67 = typedef "Config Module.lvlib/Config File Operation Enum.ctl" = enum16{"Read", "Write"}
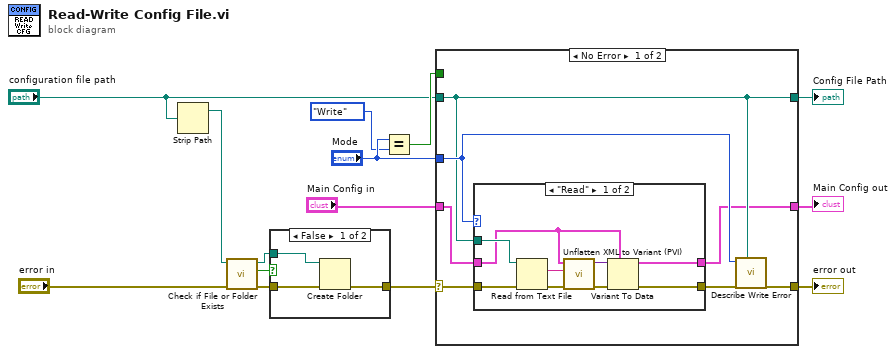
[diagram p0: block diagram]
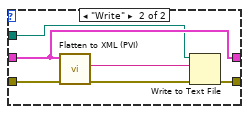
[diagram p3: hidden frame]
diagram:
  n1 = Strip Path(path="configuration file path") -> (stripped path=w9:path)  [unwired: 1 out]
  n2 = call <vilib>:"Check if File or Folder Exists.vi"("error in (no error)"="error in", "path"=w9) -> ("error out"=w6:errorcluster, "file or folder exists?"=w7:bool, "dup path"=w4:path)  [unwired: 7 in]
  n3 = case shown="False" w7 {
    tunnel: w6 -> [w17 w18]
    tunnel: [w16 w18] -> w5
    tunnel: w4 -> [w15 _]
    frame False {
      n4 = Create Folder(path (use dialog)=w15, error in=w17) -> (error out=w16:errorcluster)  [unwired: 1 in, 2 out]
    }
    frame True {
    }
  }
  n5 = Equal?(x="Mode", y=Config_File_Operation_Enum."Write" ("Mode")) -> (x = y?=w10:bool)
  n6 = case shown="No Error" w5 {
    selector: w5 -> [w21 w42]
    tunnel: [w25 w42] -> w14
    tunnel: "configuration file path" -> [w22 w43]
    tunnel: "Main Config in" -> [w23 w41]
    tunnel: [w22 w43] -> w13
    tunnel: "Mode" -> [w24 _]
    tunnel: w10 -> [_ _]
    tunnel: [w19 w41] -> w1
    frame No Error {
      n7 = case shown="\"Read\"" w24 {
        tunnel: [w28 w39] -> w19
        tunnel: w23 -> [w30 w39]
        tunnel: w21 -> [w33 w40]
        tunnel: w22 -> [w34 w37]
        tunnel: [w26 w36] -> w20
        frame "Read" {
          n8 = Read from Text File(file (use dialog)=w34, error in=w33) -> (text=w31:string, error out=w32:errorcluster)  [unwired: 2 in, 2 out]
          n9 = call "Unflatten XML to Variant (PVI).vi"("error in (no error)"=w32, "XML"=w31, "Variant in (for type and default data)"=w30) -> ("error out"=w27:errorcluster, "Variant out"=w29:variant)  [unwired: 7 in]
          n10 = Variant To Data(error in=w27, type=w30, Variant=w29) -> (data=w28:T1, error out=w26:errorcluster)
        }
        frame "Write" {
          n11 = call "Flatten to XML (PVI).vi"("error in (no error)"=w40, "Variant"=w39) -> ("error out"=w38:errorcluster, "XML"=w35:string)  [unwired: 8 in]
          n12 = Write to Text File(file (use dialog)=w37, text=w35, error in=w38) -> (error out=w36:errorcluster)  [unwired: 1 in, 2 out]
        }
      }
      n13 = call "Describe Write Error.vi"("Config File Path"=w22, "error in (no error)"=w20, "Mode"=w24) -> ("error out"=w25:errorcluster)  [unwired: 8 in]
    }
    frame Error {
    }
  }
  "error out" <- w14
  "Config File Path" <- w13
  "Main Config out" <- w1
